vi "_007.vi"() -> ()   [LabVIEW 2024]
panel:
  in  "stop":bool
  out "Numeric indicator":dbl
  in  "Numeric control":i32
  # "Structures :"
  # "(For Loop)"
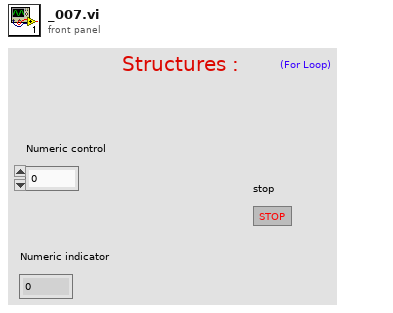
[diagram p1: front panel]
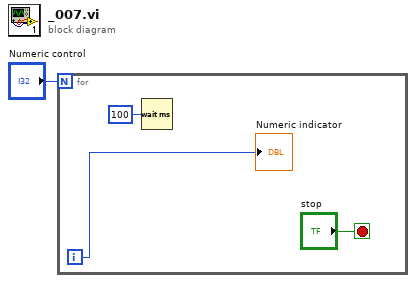
[diagram p0: block diagram]
diagram:
  n1 = for {
    N: "Numeric control" -> [_]
    i -> [w4]
    stop <- "stop" stop-if-true
    n2 = Wait (ms)(milliseconds to wait=u32 100) -> ()  [unwired: 1 out]
    "Numeric indicator" <- w4
  }
